vi "Duplicate.vi"(8 "error in (no error)":errorcluster, 10 "new Pointer type":refnum<class "Pointer.lvclass">, 11 "Pointer in":refnum<class "Pointer.lvclass">) -> (0 "error out":errorcluster, 2 "new Pointer":refnum<class "Pointer.lvclass">, 3 "Pointer out":refnum<class "Pointer.lvclass">)   [LabVIEW 2020, in "Memory Manager.lvlib" / "Pointer.lvclass"]
doc: "Allocates a new Pointer of the specified type that is the same size as <b>Pointer</b>, and copies the contents of <b>Pointer</b> to <b>new Pointer</b>."
uses:
  Pointer.lvclass
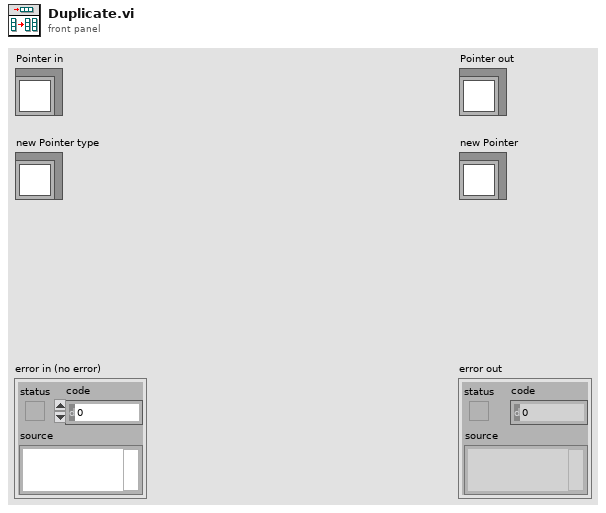
[diagram p1: front panel]
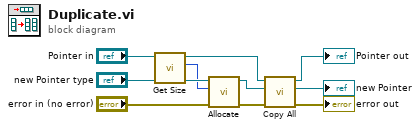
[diagram p0: block diagram]
diagram:
  n1 = call "Get Size.vi"("Pointer in"="Pointer in") -> ("size"=w2:u64, "Pointer out"=w8:refnum<class "Pointer.lvclass">)  [unwired: 9 in]
  n2 = call "Allocate.vi"("error in (no error)"="error in (no error)", "size"=w2, "Pointer type"="new Pointer type") -> ("error out"=w10:errorcluster, "Pointer out"=w9:refnum<class "Pointer.lvclass">)  [unwired: 7 in]
  n3 = call "Copy All.vi"("error in (no error)"=w10, "dst Pointer in"=w9, "src Pointer in"=w8) -> ("error out"=→"error out":errorcluster, "dst Pointer out"=→"new Pointer":refnum<class "Pointer.lvclass">, "src Pointer out"=→"Pointer out":refnum<class "Pointer.lvclass">)  [unwired: 6 in]
